vi "grabLastGrayScaleImage.vi"(0 "ImageInstance":T2, 1 "errorIn":errorcluster, 2 "AlliedVisionImageGrabPatch":bool, 3 "SessionIn":T1, 4 "bufferNumberIn":u32) -> (5 "ImageOut":T2, 6 "errorOut":errorcluster, 7 "bufferNumberActual":u32, 8 "sessionOut":T1)   [LabVIEW 2021]
uses:
  <vilib>/vision/Image Controls.llb/IMAQ Image.ctl
  <vilib>/userDefined/High Color/IMAQdx.ctl
  <vilib>/vision/Management.llb/Cast Image 2 Method.ctl
  <vilib>/vision/driver/IMAQdx.llb/IMAQdx Buffer Number Mode.ctl
  niimaqdx.dll
  <vilib>/vision/driver/NI_Vision_Acquisition_Software.lvlib
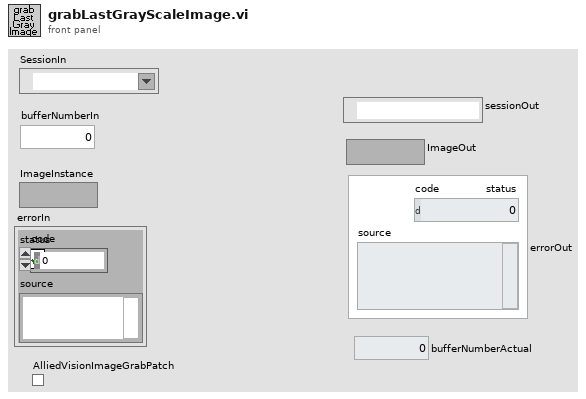
[diagram p1: front panel]
types:
  T1 = typedef "IMAQdx.ctl" = refnum<k21>
  T2 = typedef "IMAQ Image.ctl" = refnum<image>
  T3 = typedef "NI_Vision_Acquisition_Software.lvlib/IMAQdx Buffer Number Mode.ctl" = enum32{"Next", "Last", "Buffer Number", "Every", "Last New"}
  T4 = typedef "Cast Image 2 Method.ctl" = u32
  T5 = typedef "Image Type" = u32
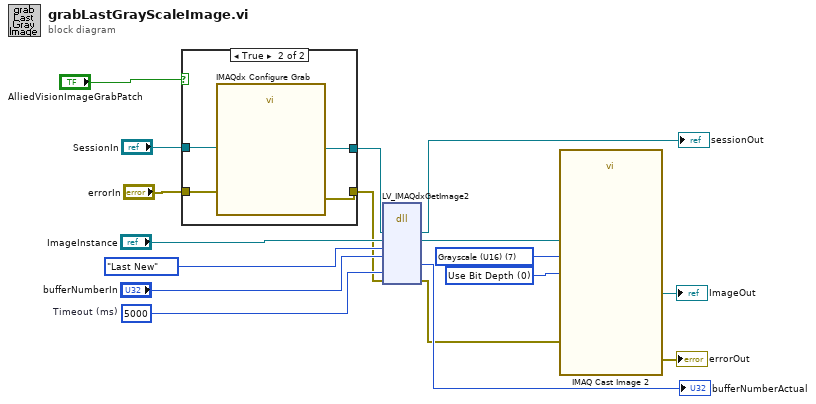
[diagram p0: block diagram]
diagram:
  w13 = 5000  # Timeout (ms)
  w16 = T4 0 items=["Use Bit Depth", "Shift", "Use Lookup Table"] ("Method")
  w15 = T5 7 items=["Grayscale (U8)", "Grayscale (I16)", "Grayscale (SGL)", "Complex (CSG)", "RGB (U32)", "HSL (U32)", "RGB (U64)", "Grayscale (U16)"] ("Image Type")
  n1 = case shown="True" "AlliedVisionImageGrabPatch" {
    tunnel: "SessionIn" -> [w19 w23]
    tunnel: [w19 w22] -> w4
    tunnel: "errorIn" -> [w18 w21]
    tunnel: [w18 w20] -> w2
    frame False {
    }
    frame True {
      n2 = call <vilib>:"IMAQdx Configure Grab.vi"("error in"=w21, "Session In"=w23) -> ("error out"=w20:errorcluster, "Session Out"=w22:T1)  [unwired: 8 in]
    }
  }
  n3 = dll-call lib="niimaqdx.dll" fn="LV_IMAQdxGetImage2"("refnum"=w4, "image"="ImageInstance", "mode"=IMAQdx_Buffer_Number_Mode."Last New" ("Buffer Number Mode"), "bufferNumberDesired"="bufferNumberIn", "timeoutMs"=w13, "error"=w2) -> ("refnum"=→"sessionOut":T1, "image"=w7:T2, "bufferNumberActual"=→"bufferNumberActual":u32, "error"=w9:errorcluster)  [unwired: 8 in, 2 out]
  n4 = call "IMAQ Cast Image 2"("Image Src"=w7, "Method"=w16, "Image Type"=w15, "error in (no error)"=w9) -> ("Image Dst Out"=→"ImageOut":T2, "error out"=→"errorOut":errorcluster)  [unwired: 10 in]
